vi "Update Running State.vi"(8 "error in (no error)":errorcluster, 10 "Is Running":bool, 11 "Plugin Session in":refnum<class "Plugin Session.lvclass">) -> (0 "error out":errorcluster, 3 "Plugin Session out":refnum<class "Plugin Session.lvclass">)   [LabVIEW 2020, in "InstrumentStudio Plugin SDK.lvlib" / "Plugin Session.lvclass"]
uses:
  Plugin Session.lvclass
  Plugin Session.lvclass/Plugin Session.ctl
  Read Session Id.vi
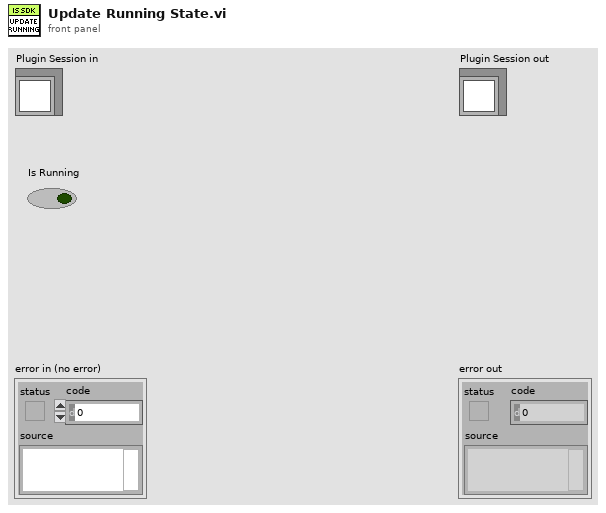
[diagram p1: front panel]
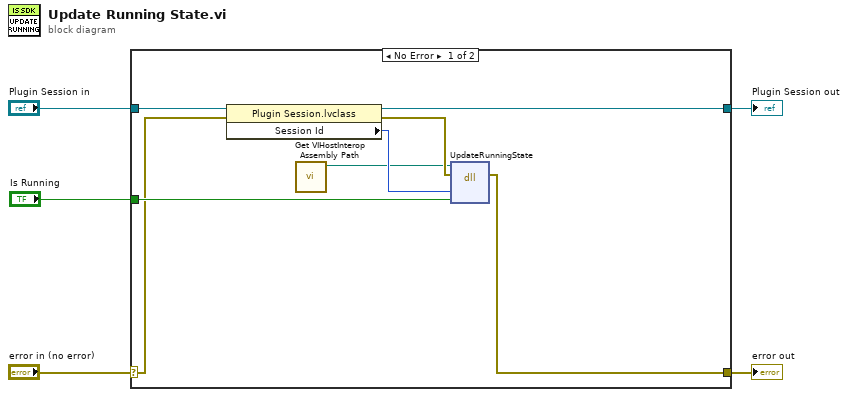
[diagram p0: block diagram]
diagram:
  n1 = case shown="No Error" "error in (no error)" {
    selector: "error in (no error)" -> [w9 w15]
    tunnel: [w7 w15] -> w4
    tunnel: [w11 w14] -> w2
    tunnel: "Plugin Session in" -> [w12 w14]
    tunnel: "Is Running" -> [w13 _]
    frame No Error {
      n2 = property class="Plugin Session.lvclass"(reference=w12, error in=w9) -> (reference out=w11:refnum<class "Plugin Session.lvclass">, error out=w8:errorcluster, "Session Id"=w10:u64)
      n3 = call "Get VIHostInterop Assembly Path.vi"() -> ("VIHost.Interop Assembly"=w6:path)  [unwired: 11 in]
      n4 = dll-call lib="C:/ASW/Source/InstrumentStudio/IFDistribution/VIHostPanel/objects/export/targets/win64U/x64/msvc-14.0/debug/NationalInstruments.VIHost.Interop.dll" fn="UpdateRunningState"(path in=w6, error in=w8, "sessionId"=w10, "isRunning"=w13) -> (error out=w7:errorcluster)  [unwired: 4 in, 1 out]
    }
    frame Error {
    }
  }
  "error out" <- w4
  "Plugin Session out" <- w2
